vi "ProcessWrapper.vi"(8 "error in (no error)":errorcluster, 11 "ConfigManager.Text in":refnum<class "ConfigManager.Text.lvclass">) -> (0 "error out":errorcluster, 3 "ConfigManager.Text out":refnum<class "ConfigManager.Text.lvclass">)   [LabVIEW 2013, in "CfgManager.Text.lvlib" / "ConfigManager.Text.lvclass"]
uses:
  ConfigManager.Text.lvclass
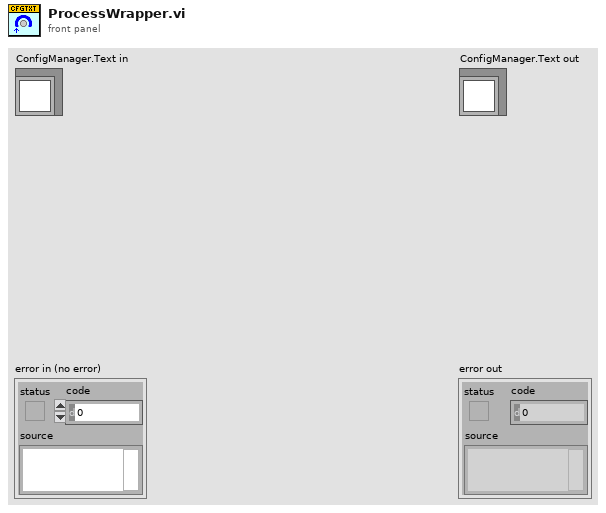
[diagram p1: front panel]
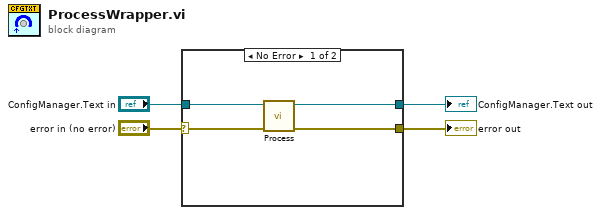
[diagram p0: block diagram]
diagram:
  n1 = case shown="No Error" "error in (no error)" {
    selector: "error in (no error)" -> [w5 w10]
    tunnel: [w6 w10] -> w3
    tunnel: [w7 w9] -> w1
    tunnel: "ConfigManager.Text in" -> [w8 w9]
    frame No Error {
      n2 = call-dynamic "Process.vi"("error in (no error)"=w5, "ConfigManager.Text in"=w8) -> ("error out"=w6:errorcluster, "ConfigManager.Text out"=w7:refnum<class "ConfigManager.Text.lvclass">)  [unwired: 8 in]
    }
    frame Error {
    }
  }
  "error out" <- w3
  "ConfigManager.Text out" <- w1
